vi "Get DATA.vi"(8 "error in":errorcluster, 11 "axis in":cluster{"keyHandle":u32, "nodeId":u16}={"keyHandle"=262145, "nodeId"=1}) -> (0 "error out":errorcluster, 3 "axis out":cluster{"keyHandle":u32, "nodeId":u16}={"keyHandle"=262145, "nodeId"=1})   [LabVIEW 2018]
panel:
  in  "Boolean":bool
  in  "Tab Control":T1(tab)=enum."Library Data"
  out "motor Data":T2={"motor Type"=1, "continuousCurrent"=0, "peakCurrent"=0, "polePair"=0, "thermalTimeConstant"=0} {"motor Type" items=["Phase modulated DC motor "=1, "Sinusoidal PM BL motor"=10, "Trapezoidal PM BL motor"=11]}
  out "encoder parameter":cluster{"sensorType":u16, "encoder counts":u32}={"sensorType"=1, "encoder counts"=0} {"sensorType" items=["Incremental Encoder (3 Channel)"=1, "Incremental Encoder (2 Channel)"=2, "Halls Sensors"=3]}
  out "Current Control Gains":cluster{"p-Gain":u16, "i-Gain":u16}
  out "Position Control Gains":T3
  out "libraryName":string="maxon motor ag - EPOS Command Library - 32-Bit"
  out "libraryVersion":string="1.0.0.0"
  out "targetReached":i32
  # "Parameter of EPOS2/4"
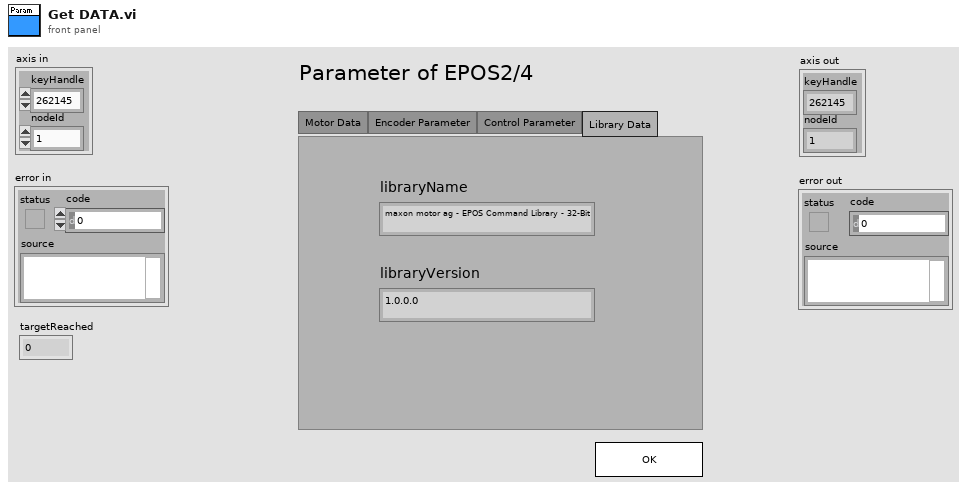
[diagram p1: front panel]
types:
  T1 = enum32{"Motor Data", "Encoder Parameter", "Control Parameter", "Library Data"}
  T2 = cluster{"motor Type":u16, "continuousCurrent":u16, "peakCurrent":u16, "polePair":u8, "thermalTimeConstant":u16}
  T3 = cluster{"p-Gain":u16, "i-Gain":u16, "d-Gain":u16}
  T4 = cluster{"nominalCurrent":u16, "maxOutputCurrent":u16, "thermalTimeConstant":u16, "nbOfPolePairs":u8}
  T5 = cluster{"motor type":u16, "nominalCurrent":u16, "maxOutputCurrent":u16, "nbOfPolePairs":u8, "thermalTimeConstant":u16}
  T6 = cluster{"nominal current":u16, "max output current":u16, "thermal time constant":u16}
  T7 = cluster{"motor type":u16, "nominal current":u16, "max output current":u16, u8, "thermal time constant":u16}
  T8 = cluster{"encoderResolution":u32, "invertedPolarity":i32}
  T9 = cluster{"sensorType":u16, "encoderResolution":u32}
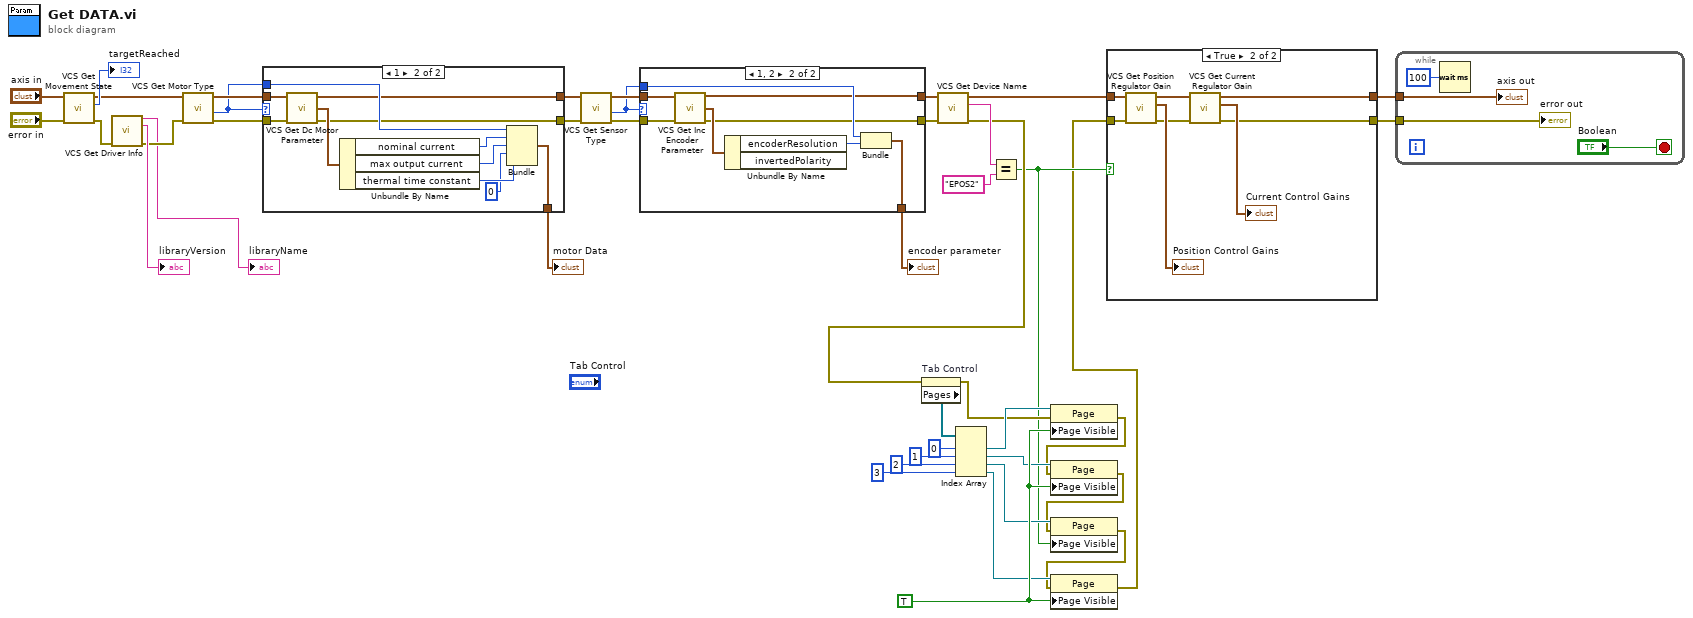
[diagram p0: block diagram]
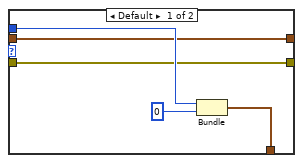
[diagram p3: hidden frame]
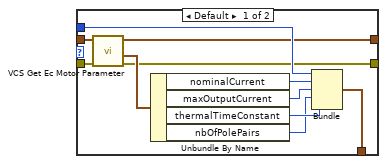
[diagram p4: hidden frame]
diagram:
  w13 = TRUE ("Page Visible")
  n1 = call "VCS Get Movement State.vi"("error in (no error)"="error in", "axis in"="axis in") -> ("error out"=w39:errorcluster, "targetReached"=→"targetReached":i32, "axis out"=w34:cluster{"keyHandle":u32, "nodeId":u16})  [unwired: 7 in]
  n2 = call "VCS Get Driver Info.vi"("error in (no error)"=w39) -> ("libraryName"=→"libraryName":string, "libraryVersion"=→"libraryVersion":string, "error out"=w35:errorcluster)  [unwired: 12 in]
  n3 = call "VCS Get Motor Type.vi"("error in (no error)"=w35, "axis in"=w34) -> ("error out"=w32:errorcluster, "motor type"=w31:u16, "axis out"=w33:cluster{"keyHandle":u32, "nodeId":u16})  [unwired: 7 in]
  n4 = case shown="1" w31 {
    tunnel: w33 -> [w53 w64]
    tunnel: w32 -> [w52 w63]
    tunnel: w31 -> [w48 w61]
    tunnel: [w47 w58] -> w30
    tunnel: [w44 w55] -> w29
    tunnel: [w43 w54] -> w28
    frame Default {
      n5 = call "VCS Get Ec Motor Parameter.vi"("error in (no error)"=w52, "axis in"=w53) -> ("error out"=w43:errorcluster, "EC motor parameter"=w49:T4, "axis out"=w44:cluster{"keyHandle":u32, "nodeId":u16})  [unwired: 3 in]
      n6 = Unbundle By Name(w49) -> ("nominalCurrent"=w51:u16, "maxOutputCurrent"=w50:u16, "thermalTimeConstant"=w46:u16, "nbOfPolePairs"=w45:u8)
      n7 = Bundle("motor type"=w48, "nominalCurrent"=w51, "maxOutputCurrent"=w50, "nbOfPolePairs"=w45, "thermalTimeConstant"=w46) -> (w47:T5)  [unwired: 1 in]
    }
    frame 1 {
      n8 = call "VCS Get Dc Motor Parameter.vi"("axis in"=w64, "error in (no error)"=w63) -> ("axis out"=w55:cluster{"keyHandle":u32, "nodeId":u16}, "DC motor parameter"=w62:T6, "error out"=w54:errorcluster)  [unwired: 11 in]
      n9 = Unbundle By Name(w62) -> ("nominal current"=w60:u16, "max output current"=w59:u16, "thermal time constant"=w57:u16)
      n10 = Bundle("motor type"=w61, "nominal current"=w60, "max output current"=w59, u8 0, "thermal time constant"=w57) -> (w58:T7)  [unwired: 1 in]
    }
  }
  "motor Data" <- w30
  n11 = call "VCS Get Sensor Type.vi"("error in (no error)"=w28, "axis in"=w29) -> ("error out"=w27:errorcluster, "sensorType"=w25:u16, "axis out"=w26:cluster{"keyHandle":u32, "nodeId":u16})  [unwired: 7 in]
  n12 = case shown="1, 2" w25 {
    tunnel: w27 -> [w65 w77]
    tunnel: w26 -> [w66 w76]
    tunnel: w25 -> [w68 w74]
    tunnel: [w69 w73] -> w24
    tunnel: [w66 w71] -> w20
    tunnel: [w65 w70] -> w22
    frame Default {
      n13 = Bundle("sensorType"=w68, u32 0) -> (w69:cluster{"sensorType":u16, u32})  [unwired: 1 in]
    }
    frame 1, 2 {
      n14 = call "VCS Get Inc Encoder Parameter.vi"("axis in"=w76, "error in (no error)"=w77) -> ("axis out"=w71:cluster{"keyHandle":u32, "nodeId":u16}, "incremental encoder parameter"=w75:T8, "error out"=w70:errorcluster)  [unwired: 11 in]
      n15 = Unbundle By Name(w75) -> ("encoderResolution"=w72:u32)  [unwired: 1 out]
      n16 = Bundle("sensorType"=w74, "encoderResolution"=w72) -> (w73:T9)  [unwired: 1 in]
    }
  }
  "encoder parameter" <- w24
  n17 = call "VCS Get Device Name.vi"("error in (no error)"=w22, "axis in"=w20) -> ("error out"=w3:errorcluster, "deviceName"=w18:string, "axis out"=w21:cluster{"keyHandle":u32, "nodeId":u16})  [unwired: 7 in]
  n18 = property on="Tab Control" class="TabCtl (strict)"(error in=w3) -> (error out=w7:errorcluster, "Pages"=w11:refnum<vi>[])  [unwired: 1 in, 1 out]
  n19 = Index Array(array=w11, index #1=0 ("index"), index #2=1 ("index"), index #3=2 ("index"), index #4=3 ("index")) -> (element #1=w12:refnum<vi>, element #2=w10:refnum<vi>, element #3=w9:refnum<vi>, element #4=w8:refnum<vi>)
  n20 = Equal?(x=w18, y="EPOS2" ("x")) -> (x = y?=w2:bool)
  n21 = property class="Page"(reference=w12, error in=w7, "Page Visible"=w13) -> (error out=w6:errorcluster)  [unwired: 1 out]
  n22 = property class="Page"(reference=w10, error in=w6, "Page Visible"=w13) -> (error out=w5:errorcluster)  [unwired: 1 out]
  n23 = property class="Page"(reference=w9, error in=w5, "Page Visible"=w2) -> (error out=w4:errorcluster)  [unwired: 1 out]
  n24 = property class="Page"(reference=w8, error in=w4, "Page Visible"=w13) -> (error out=w1:errorcluster)  [unwired: 1 out]
  n25 = case shown="True" w2 {
    tunnel: [w79 w83] -> w37
    tunnel: [w78 w82] -> w36
    tunnel: w1 -> [w78 w81]
    tunnel: w21 -> [w79 w80]
    frame False {
    }
    frame True {
      n26 = call "VCS Get Position Regulator Gain.vi"("error in (no error)"=w81, "axis in"=w80) -> ("error out"=w84:errorcluster, "gains"=→"Position Control Gains":T3, "axis out"=w85:cluster{"keyHandle":u32, "nodeId":u16})  [unwired: 7 in]
      n27 = call "VCS Get Current Regulator Gain.vi"("error in (no error)"=w84, "axis in"=w85) -> ("error out"=w82:errorcluster, "gains"=→"Current Control Gains":cluster{"p-Gain":u16, "i-Gain":u16}, "axis out"=w83:cluster{"keyHandle":u32, "nodeId":u16})  [unwired: 7 in]
    }
  }
  n28 = while {
    tunnel: w37 -> [w91]
    tunnel: w36 -> [w90]
    stop <- "Boolean" stop-if-true
    n29 = Wait (ms)(milliseconds to wait=u32 100) -> ()  [unwired: 1 out]
    "error out" <- w90
    "axis out" <- w91
  }
